vi "coordinates for simulation.vi"(0 "phi1":dbl, 5 "k1":dbl, 9 "phi2":dbl, 11 "k2":dbl, 12 "s1":dbl, 14 "s2":dbl) -> (4 "X":dbl[](array[numeric]), 8 "Y":dbl[](array[numeric]), 15 "Z":dbl[](array[numeric]))   [LabVIEW 2017]
uses:
  <vilib>/imath/engines/lvmath2/RunTimeEngine/Managers/WorkSpace/UID Generator.vi
  <vilib>/imath/engines/lvmath2/RunTimeEngine/RunTimeType/NIMS_RunTimeType_From StrictType (excl LVString).vi
  <instcachedir>/0/NIMS_RunTimeType_From StrictType (excl LVString)_1019F277F0A747EDBCA0F6C52CA54500.lvgen/NIMS_RunTimeType_From StrictType (excl LVString)_1019F277F0A747EDBCA0F6C52CA54500_000.vi
  <vilib>/imath/engines/lvmath2/RunTimeEngine/LocalVariableDefStatement/MC_LocalVariableDefStatement_Display.vi
  <vilib>/imath/engines/lvmath2/RunTimeEngine/Managers/SymbolTable/Clear UID.vi
  <vilib>/imath/engines/lvmath2/RunTimeEngine/NodeEndStatement/NIMS_NodeEndStatement_Output.vi
  <instcachedir>/0/NIMS_NodeEndStatement_Output_53EC0D466D134D7ABD903AC30B43404B.lvgen/NIMS_NodeEndStatement_Output_53EC0D466D134D7ABD903AC30B43404B_001.vi
  <vilib>/imath/engines/lvmath2/RunTimeEngine/ErrorHandling/NIMS_Finalize Error.vi
  <vilib>/imath/engines/lvmath2/RunTimeEngine/Managers/SymbolTable/NIMS_WorkSpace.lvlib
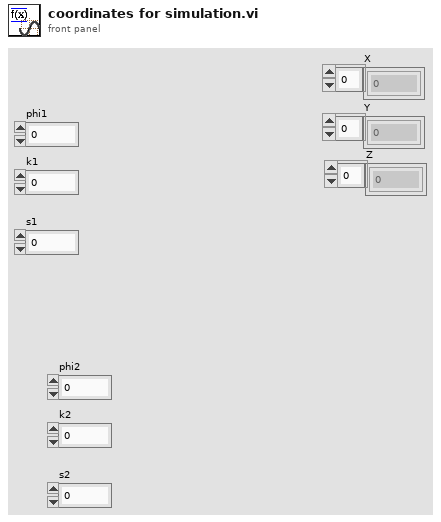
[diagram p1: front panel]
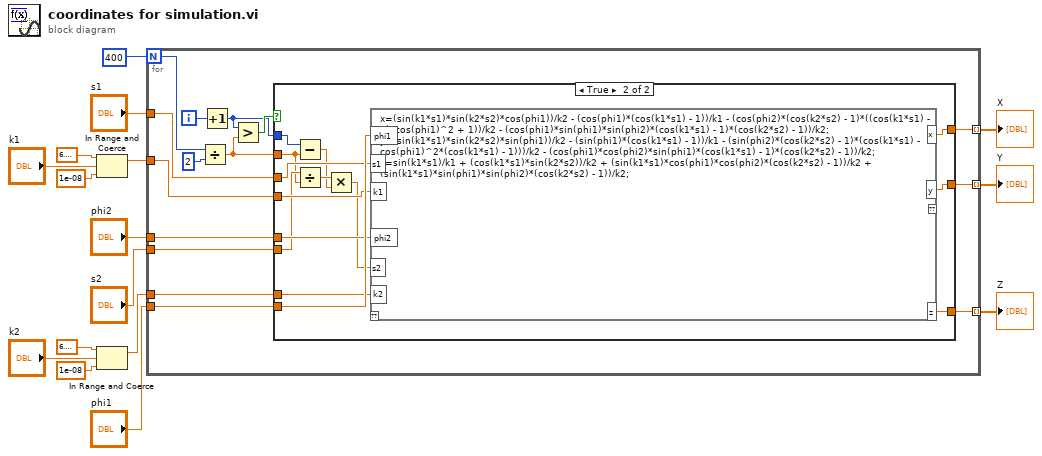
[diagram p0: block diagram]
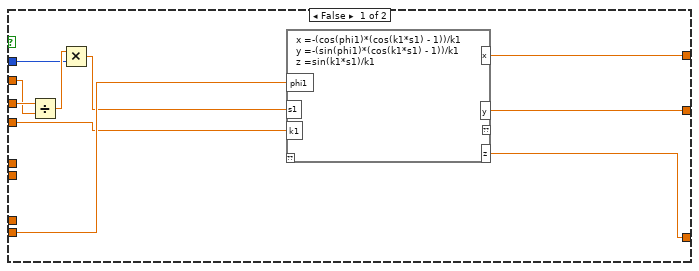
[diagram p2: hidden frame]
diagram:
  n1 = In Range and Coerce(upper limit=6.283185307179586, x="k1", lower limit=1e-08) -> (coerced(x)=w10:dbl)  [unwired: 1 out]
  n2 = In Range and Coerce(upper limit=6.283185307179586, x="k2", lower limit=1e-08) -> (coerced(x)=w2:dbl)  [unwired: 1 out]
  n3 = for {
    N: 400 -> [w22]
    tunnel: [w31] -> w15 mode=indexing
    tunnel: [w30] -> w14 mode=indexing
    tunnel: [w29] -> w13 mode=indexing
    tunnel: "phi1" -> [w28]
    tunnel: "s1" -> [w23]
    tunnel: w10 -> [w27]
    tunnel: "phi2" -> [w19]
    tunnel: w2 -> [w18]
    tunnel: "s2" -> [w17]
    i -> [w25]
    n4 = Divide(x=w22, y=2) -> (x/y=w20:dbl)
    n5 = Increment(x=w25) -> (x+1=w21:i32)
    n6 = Greater?(x=w21, y=w20) -> (0:w24:bool)
    n7 = case shown="True" w24 {
      tunnel: [w39 w149] -> w31
      tunnel: [w38 w148] -> w30
      tunnel: [w37 w147] -> w29
      tunnel: w28 -> [w41 w146]
      tunnel: w27 -> [w40 w144]
      tunnel: w23 -> [w36 w145]
      tunnel: w21 -> [w34 w138]
      tunnel: w20 -> [w32 w136]
      tunnel: w19 -> [_ w143]
      tunnel: w18 -> [_ w142]
      tunnel: w17 -> [_ w141]
      frame False {
        n8 = Divide(x=w36, y=w32) -> (x/y=w35:dbl)
        n9 = Multiply(x=w35, y=w34) -> (x*y=w33:dbl)
        n10 = mathscript code="x =-(cos(phi1)*(cos(k1*s1) - 1))/k1\ny =-(sin(phi1)*(cos(k1*s1) - 1))/k1\nz =sin(k1*s1)/k1"("phi1"=w41, "s1"=w33, "k1"=w40) -> ("x"=w39:dbl, "y"=w38:dbl, "z"=w37:dbl)  [unwired: 1 in, 1 out]
      }
      frame True {
        n11 = Subtract(x=w138, y=w136) -> (x-y=w137:dbl)
        n12 = Divide(x=w141, y=w136) -> (x/y=w140:dbl)
        n13 = Multiply(x=w140, y=w137) -> (x*y=w139:dbl)
        n14 = mathscript code="x=(sin(k1*s1)*sin(k2*s2)*cos(phi1))/k2 - (cos(phi1)*(cos(k1*s1) - 1))/k1 - (cos(phi2)*(cos(k2*s2) - 1)*((cos(k1*s1) - 1)*cos(phi1)^2 + 1))/k2 - (cos(phi1)*sin(phi1)*sin(phi2)*(cos(k1*s1) - 1)*(cos(k2*s2) - 1))/k2;\ny=(sin(k1*s1)*sin(k2*s2)*sin(phi1))/k2 - (sin(phi1)*(cos(k1*s1) - 1))/k1 - (sin(phi2)*(cos(k2*s2) - 1)*(cos(k1*s1) - cos(phi1)^2*(cos(k1*s1) - 1)))/k2 - (cos(phi1)*cos(phi2)*sin(phi1)*(cos(k1*s1) - 1)*(cos(k2*s2) - 1))/k2;\nz=sin(k1*s1)/k1 + (cos(k1*s1)*sin(k2*s2))/k2 + (sin(k1*s1)*cos(phi1)*cos(phi2)*(cos(k2*s2) - 1))/k2 + (sin(k1*s1)*sin(phi1)*sin(phi2)*(cos(k2*s2) - 1))/k2;"("phi1"=w146, "s1"=w145, "k1"=w144, "phi2"=w143, "s2"=w139, "k2"=w142) -> ("x"=w149:dbl, "y"=w148:dbl, "z"=w147:dbl)  [unwired: 1 in, 1 out]
      }
    }
  }
  "X" <- w15
  "Y" <- w14
  "Z" <- w13
